vi "LXM32_Close.vi"(8 "error in":errorcluster, 11 "VISA resource name":refnum<visa-resource-name>) -> (0 "error out":errorcluster)   [LabVIEW 2015, in "LXM32_Modbus_Serial.lvlib"]
uses:
  LXM32_Modbus_Serial.lvlib
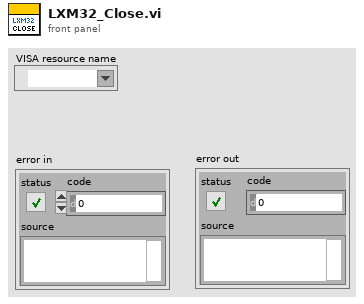
[diagram p1: front panel]
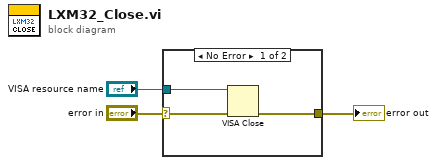
[diagram p0: block diagram]
diagram:
  n1 = case shown="No Error" "error in" {
    selector: "error in" -> [w5 w7]
    tunnel: "VISA resource name" -> [w6 _]
    tunnel: [w4 w7] -> w1
    frame No Error {
      n2 = VISA Close(VISA resource name=w6, error in (no error)=w5) -> (error out=w4:errorcluster)
    }
    frame Error {
    }
  }
  "error out" <- w1
